vi "Boiler Controller.vi"(8 "error in":errorcluster, 10 "Notifiers":T1, 11 "Message Queues":T2) -> (0 "error out":errorcluster)   [LabVIEW 2015]
uses:
  support/Message Queue/All Message Queues.ctl
  support/Message Queue/Message Cluster.ctl
  support/Notifiers/Notifiers.ctl
  support/Message Queue/Message Queue.lvlib
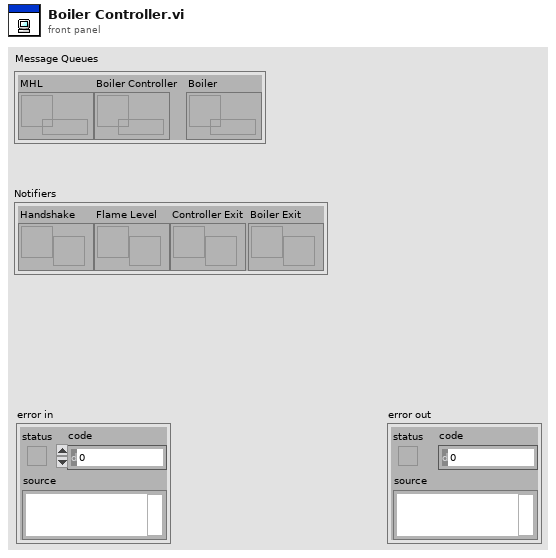
[diagram p1: front panel]
types:
  T1 = typedef "Notifiers.ctl" = cluster{"Handshake":refnum<notifier>, "Flame Level":refnum<notifier>, "Controller Exit":refnum<notifier>, "Boiler Exit":refnum<notifier>}
  T2 = typedef "Message Queue.lvlib/All Message Queues.ctl" = cluster{"MHL":refnum<queue>, "Boiler Controller":refnum<queue>, "Boiler":refnum<queue>}
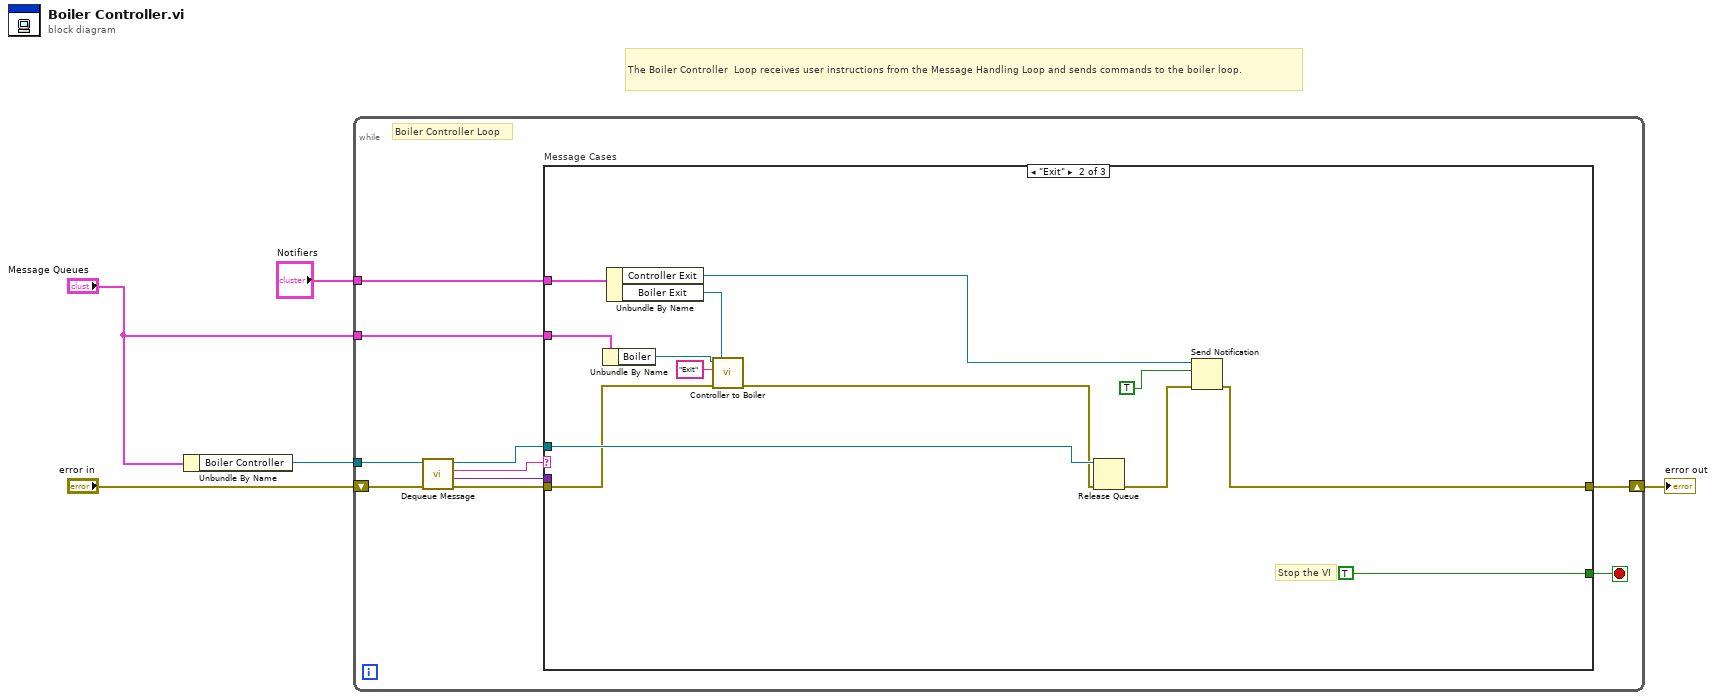
[diagram p0: block diagram]
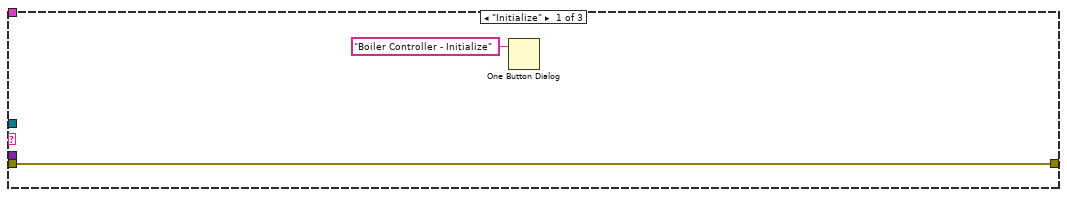
[diagram p2: hidden frame]
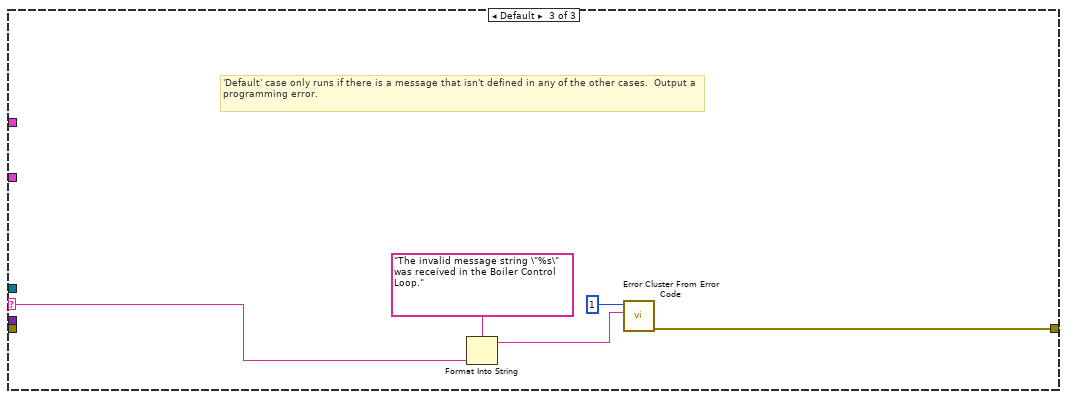
[diagram p3: hidden frame]
diagram:
  # "The Boiler Controller  Loop receives user instructions from the Message Handling Loop and sends commands to the boiler loop."
  n1 = Unbundle By Name("Message Queues") -> ("Boiler Controller"=w3:refnum<queue>)
  n2 = while {
    tunnel: w3 -> [w9]
    shift-right: [w8] -> w5
    shift-left: "error in" -> [w14]
    tunnel: "Notifiers" -> [w7]
    tunnel: "Message Queues" -> [w6]
    stop <- w15 stop-if-true
    # "Boiler Controller Loop"
    n3 = call "Dequeue Message.vi"("error in (no error)"=w14, "Message Queue"=w9) -> ("error out"=w13:errorcluster, "Message Data"=w11:variant, "Message"=w12:string, "dup Message Queue"=w10:refnum<queue>)  [unwired: 6 in]
    n4 = case "Message Cases" shown="\"Exit\"" w12 {
      selector: w12 -> [_ _ w32]
      tunnel: w10 -> [_ w29 _]
      tunnel: w13 -> [w17 w23 _]
      tunnel: [w17 w18 w31] -> w8
      tunnel: [_ TRUE _] -> w15
      tunnel: w11 -> [_ _ _]
      tunnel: w7 -> [_ w28 _]
      tunnel: w6 -> [_ w26 _]
      frame "Initialize" {
        n5 = One Button Dialog(message="Boiler Controller - Initialize") -> ()  [unwired: 1 in, 1 out]
      }
      frame "Exit" {
        # "Stop the VI"
        n6 = Unbundle By Name(w26) -> ("Boiler"=w25:refnum<queue>)
        n7 = Unbundle By Name(w28) -> ("Controller Exit"=w21:refnum<notifier>, "Boiler Exit"=w27:refnum<notifier>)
        n8 = call "Controller to Boiler.vi"("Notifier"=w27, "error in"=w23, "Message"="Exit", "Boiler Queue in"=w25) -> ("error out"=w22:errorcluster)  [unwired: 5 in, 2 out]
        n9 = Release Queue(queue=w29, error in (no error)=w22) -> (error out=w19:errorcluster)  [unwired: 1 in, 2 out]
        n10 = Send Notification(notification=TRUE, notifier=w21, error in (no error)=w19) -> (error out=w18:errorcluster)  [unwired: 1 out]
      }
      frame Default {
        # "'Default' case only runs if there is a message that isn't defined in any of the other cases.  Output a programming error."
        n11 = Format Into String(format string="The invalid message string \"%s\" was received in the Boiler Control Loop." ("Unknown Message Error Text"), w32) -> (resulting string=w33:string)  [unwired: 2 in, 1 out]
        n12 = call <vilib>:"Error Cluster From Error Code.vi"("error message (\"\")"=w33, "error code (0)"=1) -> ("error out"=w31:errorcluster)  [unwired: 7 in]
      }
    }
  }
  "error out" <- w5
